vi "Multiplexer CTL test.vi"() -> ()   [LabVIEW 2014]
uses:
  Graphic/Line/Line.lvclass
  <vilib>/Utility/miscctls.llb/LVPositionTypeDef.ctl
  <userlib>/_OpenG.lib/numeric/numeric.llb/Random Number Within Range - I32__ogtk.vi
panel:
  out "diff":T1
  out "PosBool":T2
  out "PosBCk":T2
  out "Boolean":bool
  out "Picture Bckgnd":picture
  in  "Line.lvclass":refnum<class "Line.lvclass">
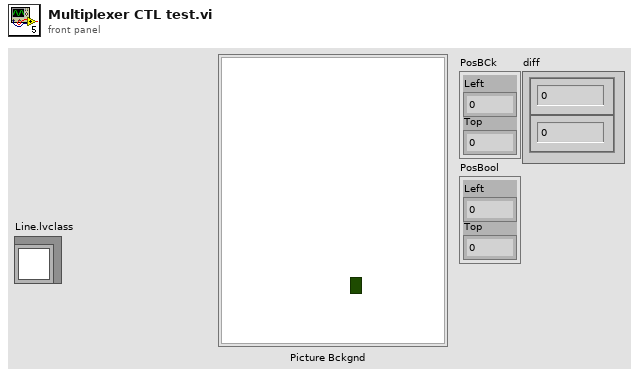
[diagram p1: front panel]
types:
  T1 = cluster{"Numeric Control":i32, "Numeric Control":i32}
  T2 = typedef "LVPositionTypeDef.ctl" = cluster{"Left":i32, "Top":i32}
  T3 = cluster{"Width":u16, "Style":enum32{"Solid", "Dash", "Dot", "DashDot", "DashDotDot"}}
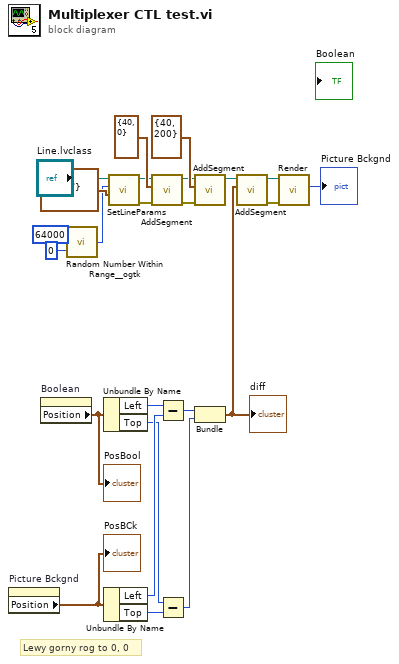
[diagram p0: block diagram]
diagram:
  # "Lewy gorny rog to 0, 0"
  n1 = property on="Picture Bckgnd" class="Pict"() -> ("Position"=w16:T2)  [unwired: 2 in, 2 out]
  "PosBCk" <- w16
  n2 = property on="Boolean" class="Bool (strict)"() -> ("Position"=w6:T2)  [unwired: 2 in, 2 out]
  "PosBool" <- w6
  n3 = call-poly <userlib>:"Random Number Within Range__ogtk.vi"("High"=64000, "Low"=0) -> ("Random Number"=w1:i32)  [unwired: 3 in]
  n4 = Unbundle By Name(w6) -> ("Left"=w7:i32, "Top"=w8:i32)
  n5 = Unbundle By Name(w16) -> ("Left"=w12:i32, "Top"=w11:i32)
  n6 = call-dynamic "SetLineParams.vi"("pen"=T3 {"Width"=20, "Style"=enum."Dash"}, "color"=w1, "Line in"="Line.lvclass") -> ("error out"=w9:errorcluster, "Line out"=w20:refnum<class "Line.lvclass">)  [unwired: 7 in]
  n7 = call-dynamic "AddSegment.vi"("error in (no error)"=w9, "point"=cluster{"x":i16, "y":i16} {"x"=40, "y"=0}, "Line in"=w20) -> ("error out"=w2:errorcluster, "Line out"=w4:refnum<class "Line.lvclass">)  [unwired: 7 in]
  n8 = Subtract(x=w7, y=w12) -> (x-y=w15:i32)
  n9 = Subtract(x=w8, y=w11) -> (x-y=w14:i32)
  n10 = call-dynamic "AddSegment.vi"("error in (no error)"=w2, "point"=cluster{"x":i16, "y":i16} {"x"=40, "y"=200}, "Line in"=w4) -> ("Line out"=w3:refnum<class "Line.lvclass">)  [unwired: 7 in, 1 out]
  n11 = Bundle(w15, w14) -> (w13:cluster{i32, i32})  [unwired: 1 in]
  "diff" <- w13
  n12 = call-dynamic "AddSegment.vi"("point"=w13, "Line in"=w3) -> ("error out"=w10:errorcluster, "Line out"=w22:refnum<class "Line.lvclass">)  [unwired: 8 in]
  n13 = call-dynamic "Render.vi"("error in (no error)"=w10, "Line in"=w22) -> ("Picture Bckgnd"=→"Picture Bckgnd":picture)  [unwired: 7 in, 2 out]
